vi "Measurement_input_panel.vi"(0 "OK":T4, 2 "setup":T5, 5 "Setup filename":string) -> (11 "Setup filename out":string, 12 "Analysis Info cluster":T8[](array[typedef])=[{"Colour"=0, "Inst type"=enum."Pitot-static tube", "Inst name"="Manometer voltage", "Symbol"="U", "Code name"="", "Extra Info"="U", "Inst Array"=enum."PWA", "Index"=0, "Voltage Index"=0, "Extra Titles"=[], "Extra Values"=[]}, {"Colour"=0, "Inst type"=enum."Pitot-static tube", "Inst name"="Manometer voltage", "Symbol"="U", "Code name"="", "Extra Info"="U", "Inst Array"=enum."PWA", "Index"=0, "Voltage Index"=0, "Extra Titles"=[], "Extra Values"=[]}, {"Colour"=0, "Inst type"=enum."Pitot-static tube", "Inst name"="Manometer voltage", "Symbol"="U", "Code name"="", "Extra Info"="U", "Inst Array"=enum."PWA", "Index"=0, "Voltage Index"=0, "Extra Titles"=[], "Extra Values"=[]}], 19 "Board type":T10=enum."Local ADAM")   [LabVIEW 2010]
uses:
  Controls/Inst_type.ctl
  Controls/Board_Types.ctl
  Controls/Analysis_info_cluster.ctl
  Controls/Instrument_Array.ctl
  Controls/Setup.ctl
  Controls/ok_button.ctl
  Controls/Trigger_Mode.ctl
  Controls/PWA_Data.ctl
  File/Setup_Filetype.ctl
  Controls/Post_Process.ctl
  Controls/App_Global.ctl
  Controls/Ch_and_Spans.ctl
  Globals/Meas_global.vi
  Globals/Trav_pos_global.vi
  Globals/LDA_meas_global_1.vi
  Globals/Preference_global.vi
panel:
  in  "Select Duplicate Channels":bool
  in  "PWA Data":T1
  out "Inst type":T2
  in  "Edit temp and Press":bool
  out "Abs Press (mbar)":dbl=1013.0 format="%.1f"
  out "Temp (deg C)":dbl=21.0 format="%.1f"
  in  "Trigger mode":T3
  in  "Select Plug Ins":bool
  in  "Sync Delay Time (ms)":dbl=24.0 format="%.2f"
  out "XW Present?":bool
  out "Read Setup File?":bool
  out "Setup Paths":string[](array[string])
  in  "Select Local ADAM Channels":bool
  out "Local ADAM Channels":string[](array[string])
  in  "stop":bool
  out "Notes":string
  in  "Setup filename selector":u16(ring) items=["Current_Setup.xls", "pitot_1.xls", "Calib_Setup.xls"]
  in  "Synchronise Analogue channels with LDA":bool
  in  "LDA set up":T6={"dimensions"=enum."2D", "Arrival spacing"=FALSE, "Transit time"=FALSE}
  in  "LDA data":enum16{"No LDA data", "Take LDA data"}(ring)=enum."Take LDA data"
  in  "Cross wire":T7(ring)
  in  "Acquisition Method":T10=enum."Local ADAM"
  in  "No of Analogue inst":i32=1
  in  "Ch & spans choices":T11(array[cluster]) {"D" format="%.2f"; "Ch No" min=0; "low limit" min=-10 max=10 format="%.2f"; "high limit" min=-10 max=10 format="%.2f"}
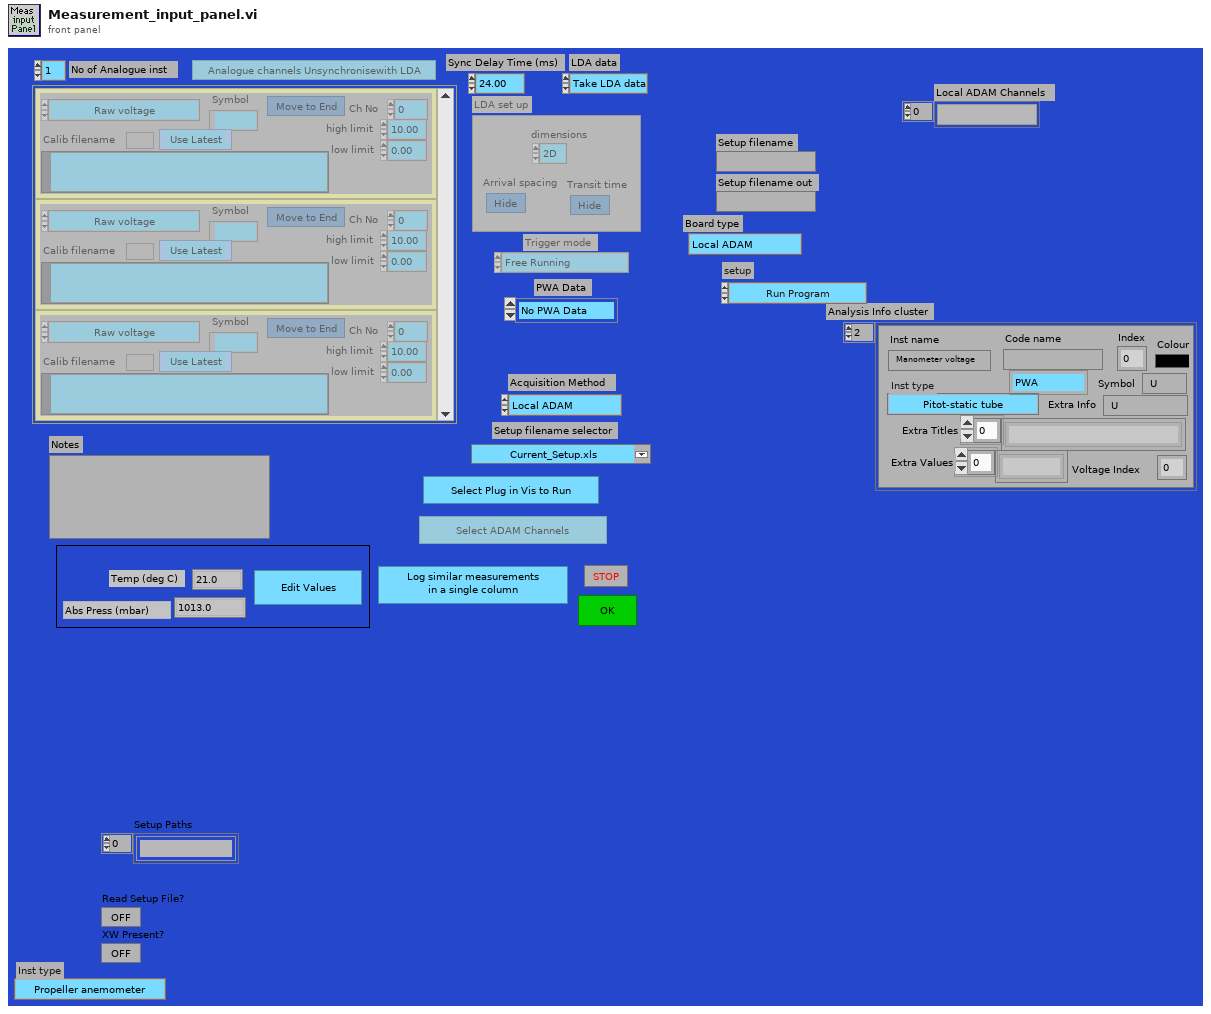
[diagram p1: front panel]
types:
  T1 = typedef "PWA_Data.ctl" = enum16{"No PWA Data", "One Ch PWA"}
  T2 = typedef "Inst_type.ctl" = enum16{"Propeller anemometer", "Raw voltage", "Pressure Transducer", "Pitot-static tube", "Preston tube", "Hot wire", "Cross wire 1", "Cross wire 2", "Generic Linear", "Generic Polynomial", "Generic BackPoly", "Fast FID", "Thermocouple", "Cold wire", "Pulsed Wire", "LDA Vel", "LDA Tran time", "LDA Arr time"}
  T3 = typedef "Trigger_Mode.ctl" = enum16{"Free Running", "Start on Trigger", "Trigger Every Block", "Trigger Every Sample"}
  T4 = typedef "ok_button.ctl" = bool
  T5 = typedef "Setup.ctl" = enum16{"Run Program", "Show Setup", "Save Current Setup", "Setup Front Panel"}
  T6 = cluster{"dimensions":enum16{"1D", "2D"}, "Arrival spacing":bool, "Transit time":bool}
  T7 = enum16{"2nd component as calculated", "2nd component multipled by -1"}
  T8 = typedef "Analysis_info_cluster.ctl" = cluster{"Colour":u32, "Inst type":T2, "Inst name":string, "Symbol":string, "Code name":string, "Extra Info":string, "Inst Array":T9, "Index":i32, "Voltage Index":i32, "Extra Titles":string[], "Extra Values":string[]}
  T9 = typedef "Instrument_Array.ctl" = enum16{"PWA", "LDA", "Analogue"}
  T10 = typedef "Board_Types.ctl" = enum16{"Simulate", "Local ADAM", "Server ADAM", "NI-DAQmx", "NI-DAQmxBase", "ADC488", "DT LV-link"}
  T11 = cluster{"high limit":sgl, "low limit":sgl, "Ch No":i16, "Calib filename":path, "Inst type":T2, "Symbol":string, "Move channel":bool, "Use Latest":bool, "D":dbl, "Ch Name":string}[]
  T12 = typedef "Post_Process.ctl" = enum16{"Take New Data", "Post Process Raw Data File"}
  T13 = typedef "Setup_Filetype.ctl" = enum16{"Measurement Setups", "Calibration Setups", "General", "Results File Plotter Setups", "Speed Calib Tweaks"}
  T14 = cluster{"high limit (10V)":sgl, "low limit (-10V)":sgl, "Ch No":i16, "Calib filename":path, "Inst type":T2, "Symbol":string, "Move channel":bool, "Use Latest":bool, "D":dbl, "Ch Name":string}
  T15 = typedef "App_Global.ctl" = enum16{"Read Global", "Write to Global", "Initialise Array"}
  T16 = typedef "Ch_and_Spans.ctl" = cluster{"high limit (10V)":sgl, "low limit (-10V)":sgl, "Ch No":i16, "Var name":string, "Use Latest Calib":bool}
  T17 = enum16{"Zero or one", "One", "Zero or more", "One or more"}
  T18 = enum8{"Enabled", "Disabled", "Disabled and Grayed Out"}
  T19 = typedef "Traverse_cluster.ctl" = cluster{"Start X":dbl, "Start Y":dbl, "Start Z":dbl, "End X":dbl, "End Y":dbl, "End Z":dbl, "No. of pts.":i32, "Spacing":T20, "Filename":path, "Tunnel Speed":dbl, "Averaging time (min)":dbl, "Extra Commands":string, "Specific Arguments":string, "Emission Rate (l/min)":dbl, "Trace Gas Concentration (%)":dbl, "Density Ratio":string, "Comments":string, "Row No":i32, "Row Type Selector":T21, "Completion time":string, "Row Duration (mins)":dbl, "No. of Valid pts.":i32, "Meas Setup File":string}
  T20 = typedef "Spacing.ctl" = enum16{"Linear", "Log", "Gauss", "Specified", "N/A"}
  T21 = typedef "Multi_run_mode.ctl" = enum16{"Move Traverse Only", "Set Tunnel Speed Only", "Set Source Only", "Set Measurement Conditions", "Single Measurement", "Vertical Profile", "Lateral Profile", "Longitudinal Profile", "Explore Volume", "Multi-Axis Profile", "Auto Calibrate", "Meas Fast FID Bkgnd", "Check Beam Power", "Scanning Valve Measurement", "Run VI Named:", "Set ADAM Ch", "Wait (minutes)", "Send Message", "Synchronize With:", "Fall Back to this Row", "Turn Off Row Repeating", "Blank Row"}
  T22 = cluster{"high limit (10V)":sgl, "low limit (-10V)":sgl, "Ch No":i16, "Calib filename":path, "Inst type":T2, "Symbol":string, "Move channel":bool, "Use Latest":bool, "D":dbl, "Ch Name":string}[]
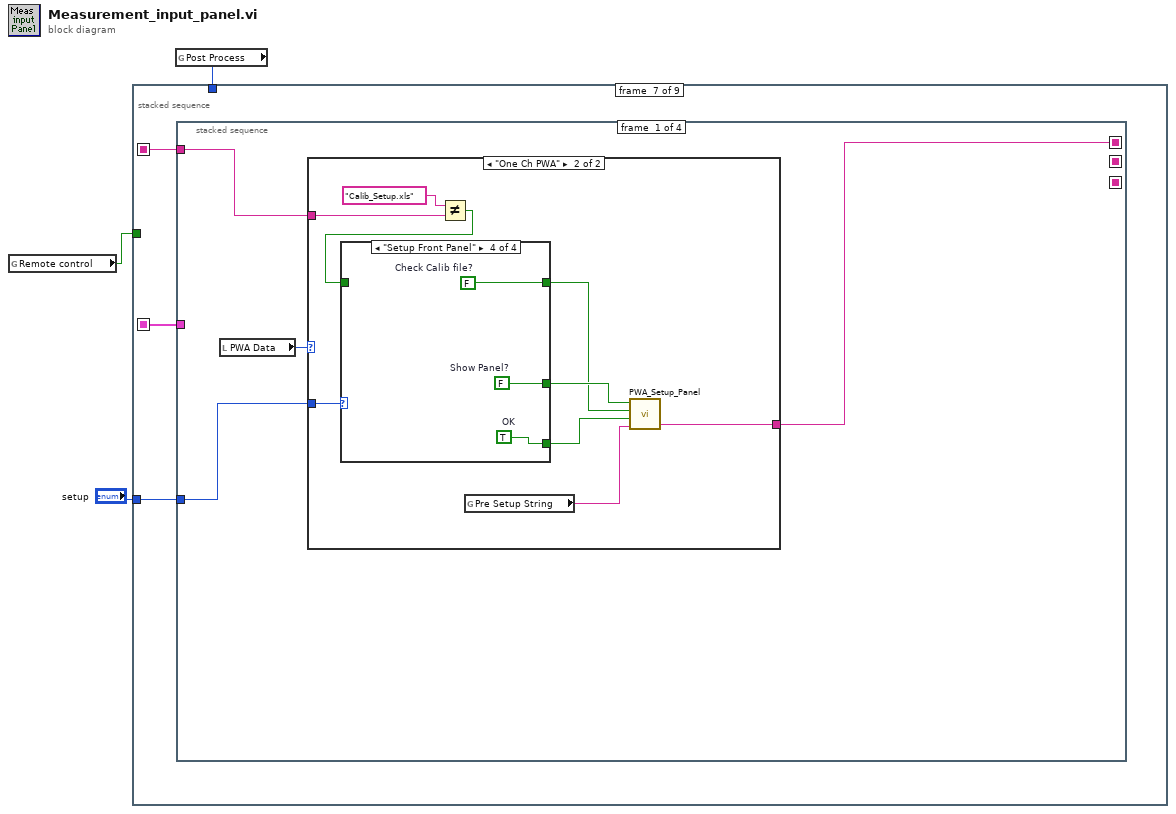
[diagram p0: block diagram]
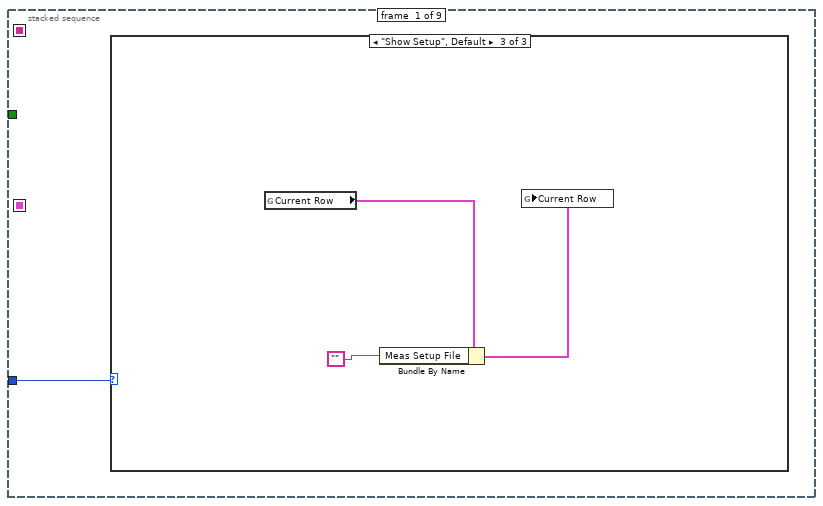
[diagram p2: hidden frame]
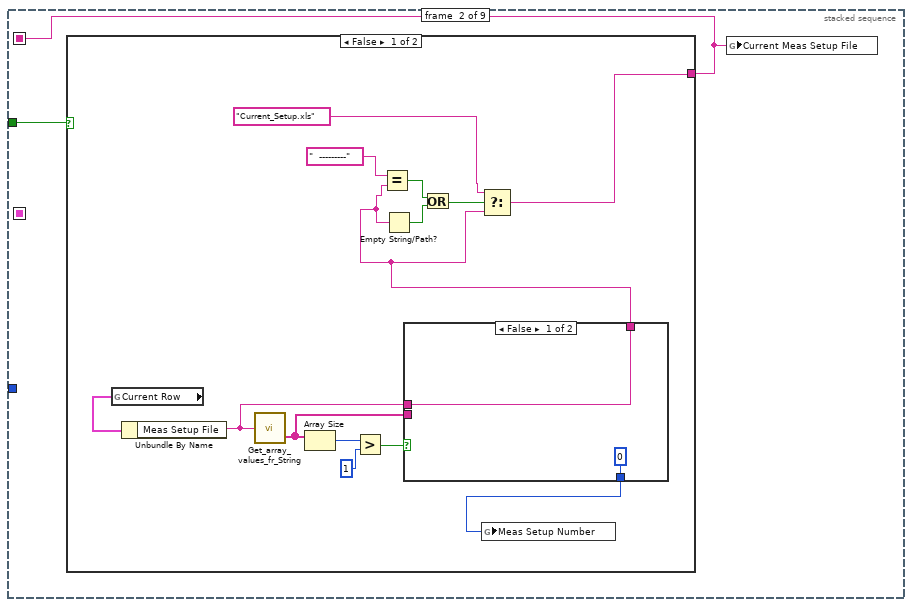
[diagram p5: hidden frame]
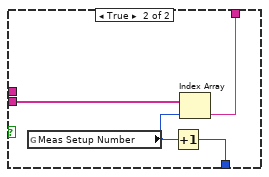
[diagram p6: hidden frame]
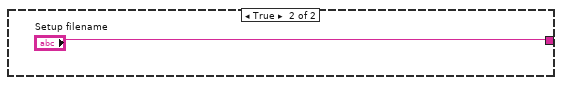
[diagram p7: hidden frame]
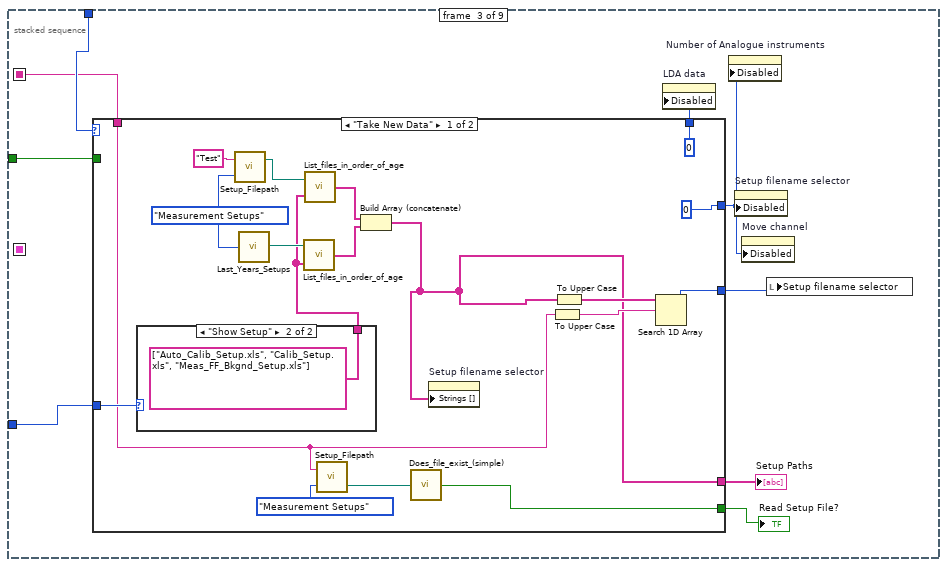
[diagram p8: hidden frame]
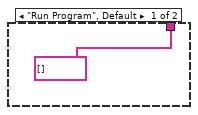
[diagram p9: hidden frame]
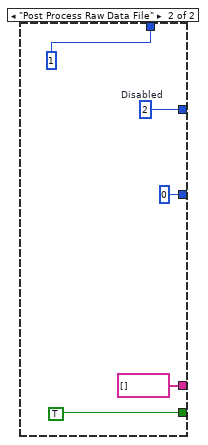
[diagram p10: hidden frame]
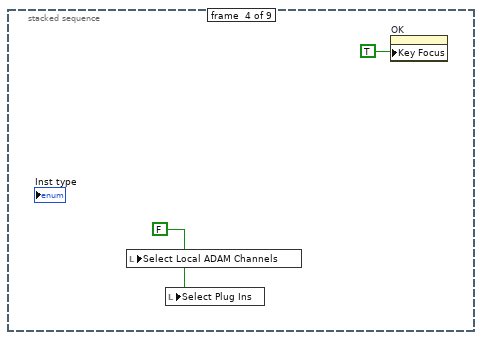
[diagram p11: hidden frame]
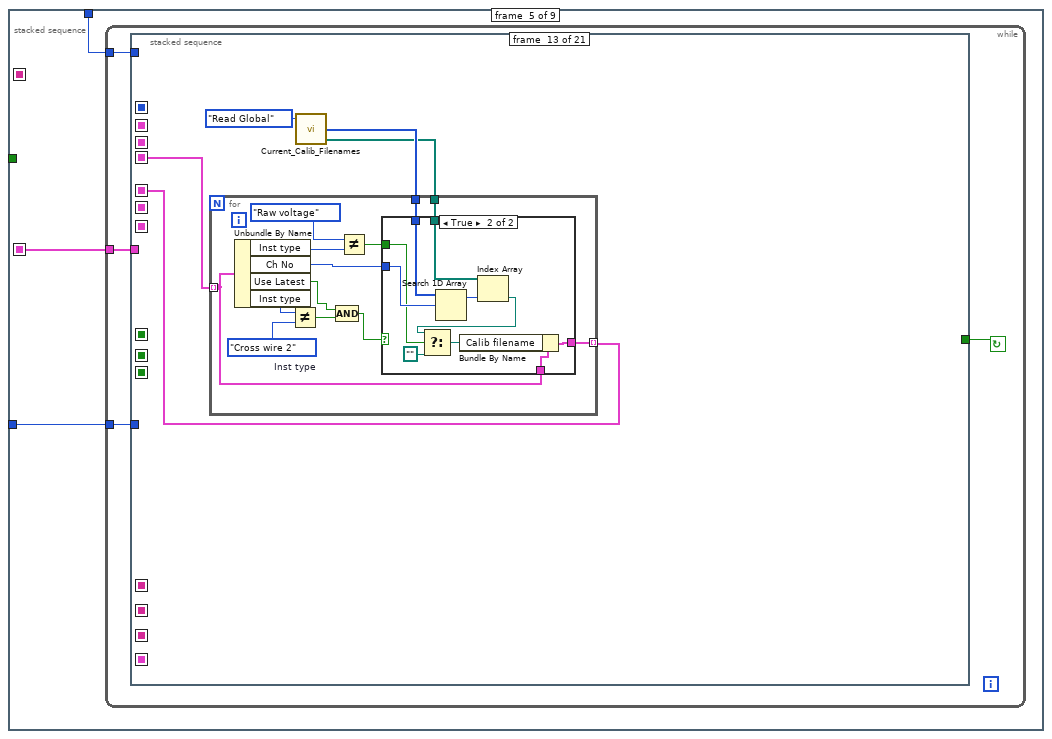
[diagram p12: hidden frame]
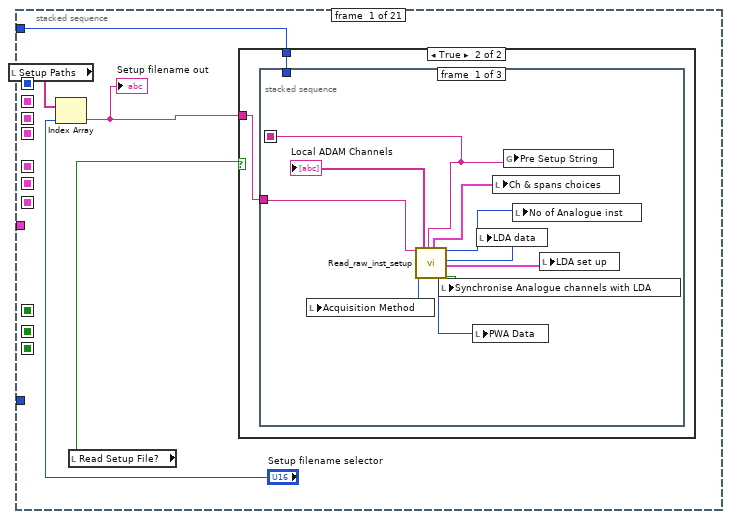
[diagram p13: hidden frame]
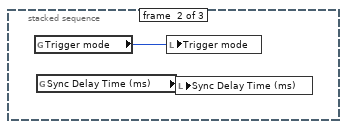
[diagram p15: hidden frame]
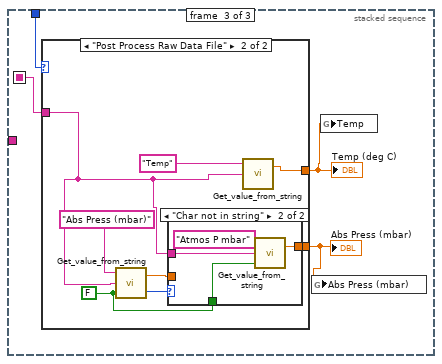
[diagram p16: hidden frame]
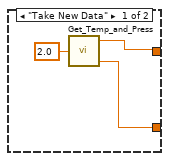
[diagram p17: hidden frame]
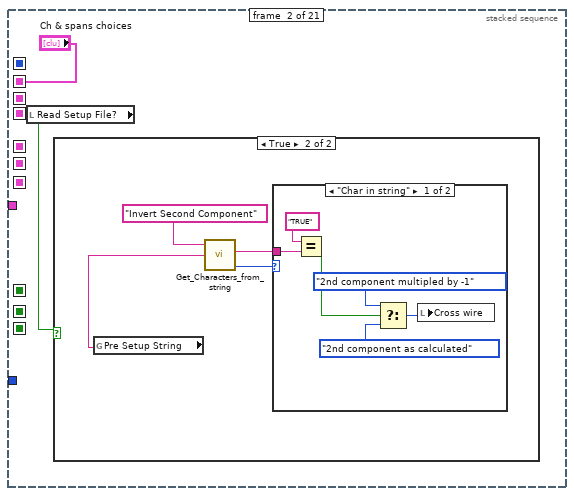
[diagram p19: hidden frame]
diagram:
  n1 = global read "Meas_global.vi" "Remote control"() -> (w1:bool)
  n2 = global read "Meas_global.vi" "Post Process"() -> (w3:T12)
  n3 = stacked-sequence {
    seq-local: [_ _ _ _ w69 _ _ _ _] -> [_ _ _ _ _ _ w723 _ w847]
    seq-local: [_ w8 _ _ _ _ _ _ _] -> [_ _ w31 _ _ _ w722 _ _]
    tunnel: w3 -> [_ _ w39 _ w68 _ _ _ w846]
    tunnel: "setup" -> [w4 _ w33 _ w67 _ w724 _ _]
    tunnel: w1 -> [_ w9 w32 _ _ _ _ _ _]
    frame #0 {
      n4 = case shown="\"Show Setup\", Default" w4 {
        frame "Run Program" {
        }
        frame "Setup Front Panel" {
        }
        frame "Show Setup", Default {
          n5 = global read "Trav_pos_global.vi" "Current Row"() -> (w7:T19)
          n6 = Bundle By Name(cluster=w7, "Meas Setup File"="") -> (w6:T19)
          n7 = global write "Trav_pos_global.vi" "Current Row"(w6) -> ()
        }
      }
    }
    frame #1 {
      n8 = case shown="False" w9 {
        tunnel: [w22 "Setup filename"] -> w8
        frame False {
          n9 = global read "Trav_pos_global.vi" "Current Row"() -> (w18:T19)
          n10 = Unbundle By Name(w18) -> ("Meas Setup File"=w12:string)
          n11 = call "Get_array_values_fr_String.vi"("String Value"=w12) -> ("String array"=w11:string[])  [unwired: 1 out]
          n12 = Array Size(array=w11) -> (size(s)=w16:i32)
          n13 = Greater?(x=w16, y=1) -> (0:w14:bool)
          n14 = case shown="False" w14 {
            tunnel: [w25 w28] -> w13
            tunnel: w12 -> [w25 _]
            tunnel: w11 -> [_ w29]
            tunnel: [0 w26] -> w10
            frame False {
            }
            frame True {
              n15 = global read "Trav_pos_global.vi" "Meas Setup Number"() -> (w27:i32)
              n16 = Increment(x=w27) -> (x+1=w26:i32)
              n17 = Index Array(array=w29, index=w27) -> (element=w28:string)
            }
          }
          n18 = Equal?(x="  ---------" ("f"), y=w13) -> (x = y?=w21:bool)
          n19 = Empty String/Path?(string/path=w13) -> (empty?=w20:bool)
          n20 = Or(x=w21, y=w20) -> (x .or. y?=w17:bool)
          n21 = Select(t="Current_Setup.xls", s=w17, f=w13) -> (s? t:f=w22:string)
          n22 = global write "Trav_pos_global.vi" "Meas Setup Number"(w10) -> ()
        }
        frame True {
        }
      }
      n23 = global write "Trav_pos_global.vi" "Current Meas Setup File"(w8) -> ()
    }
    frame #2 {
      n24 = case shown="\"Take New Data\"" w39 {
        tunnel: [w40 string[] []] -> w35
        tunnel: [w53 TRUE ("exists")] -> w34
        tunnel: [u8 0 ("Disabled") w61] -> w36
        tunnel: [u8 0 ("Disabled") u8 1 ("Disabled")] -> w38
        tunnel: w31 -> [w49 _]
        tunnel: [w56 0 ("index of element")] -> w37
        tunnel: w33 -> [w51 _]
        tunnel: w32 -> [_ _]
        frame "Take New Data" {
          w43 = Setup_Filetype."Measurement Setups" ("Setup File Type")
          n25 = case shown="\"Show Setup\"" w51 {
            tunnel: [string[] [] ("file names") string[] ["Auto_Calib_Setup.xls", "Calib_Setup.xls", "Meas_FF_Bkgnd_Setup.xls"] ("file names")] -> w41
            frame "Run Program", Default {
            }
            frame "Show Setup" {
            }
          }
          n26 = call "Setup_Filepath.vi"("Setup File Type"=w43, "Filename in"="Test") -> ("Directory"=w44:path)  [unwired: 1 out]
          n27 = call "Last_Years_Setups.vi"("Setup File Type"=w43) -> ("Directory"=w42:path)
          n28 = call "List_files_in_order_of_age.vi"("Files to Hide"=w41, "Folder"=w42) -> ("file names"=w46:string[])
          n29 = call "List_files_in_order_of_age.vi"("Files to Hide"=w41, "Folder"=w44) -> ("file names"=w45:string[])
          n30 = call "Setup_Filepath.vi"("Setup File Type"=Setup_Filetype."Measurement Setups", "Filename in"=w49) -> ("Filename Out"=w48:path)  [unwired: 1 out]
          n31 = Build Array (concatenate)(w45, w46) -> (w40:string[])
          n32 = call "Does_file_exist_(simple).vi"("Pathname"=w48) -> ("exists?"=w53:bool)
          n33 = property on="Setup filename selector" class="Ring (strict)"("Strings []"=w40) -> ()  [unwired: 2 in, 2 out]
          n34 = To Upper Case(1:w49) -> (0:w54:string)
          n35 = To Upper Case(1:w40) -> (0:w55:string[])
          n36 = Search 1D Array(1D array=w55, element=w54) -> (index of element=w56:i32)  [unwired: 1 out]
        }
        frame "Post Process Raw Data File" {
          w61 = u8 2  # Disabled
        }
      }
      "Setup Paths" <- w35
      "Read Setup File?" <- w34
      n37 = property on="LDA data" class="Enum (strict)"("Disabled"=w38) -> ()  [unwired: 2 in, 2 out]
      n38 = property on="Number of Analogue instruments" class="DigNum (strict)"("Disabled"=w36) -> ()  [unwired: 2 in, 2 out]
      n39 = property on="Setup filename selector" class="Ring (strict)"("Disabled"=w36) -> ()  [unwired: 2 in, 2 out]
      n40 = property on="Move channel" class="Bool (strict)"("Disabled"=w36) -> ()  [unwired: 2 in, 2 out]
      n41 = local write "Setup filename selector"(w37) -> ()
    }
    frame #3 {
      w66 = FALSE ("Select Local ADAM Channels")
      n42 = local write "Select Local ADAM Channels"(w66) -> ()
      n43 = local write "Select Plug Ins"(w66) -> ()
      n44 = property on="OK" class="Bool"("Key Focus"=TRUE) -> ()  [unwired: 2 in, 2 out]
    }
    frame #4 {
      n45 = while {
        tunnel: w67 -> [w70]
        tunnel: w68 -> [w71]
        tunnel: [w73] -> w69
        stop <- w72 continue-if-true
        n46 = stacked-sequence {
          seq-local: [_ _ _ _ _ _ _ _ w258 _ _ _ _ _ _ _ _ _ _ _ _] -> [_ _ _ _ _ _ _ _ _ _ w331 w376 w421 _ _ _ _ _ _ _ _]
          seq-local: [_ _ _ w147 _ _ _ _ _ _ _ _ _ _ _ _ _ _ _ _ _] -> [_ _ _ _ _ w200 w235 w254 w259 _ _ _ _ _ _ _ _ _ _ _ _]
          seq-local: [_ _ _ _ _ w205 _ _ _ _ _ _ _ _ _ _ _ _ _ _ _] -> [_ _ _ _ _ _ _ _ w260 _ _ _ _ _ _ _ _ _ _ _ _]
          seq-local: [_ _ _ _ _ _ _ _ _ _ w333 _ _ _ _ _ _ _ _ _ _] -> [_ _ _ _ _ _ _ _ _ _ _ w378 _ _ _ _ _ _ _ _ w684]
          seq-local: [_ _ _ _ _ _ _ _ _ _ _ _ _ w454 _ _ _ _ _ _ _] -> [_ _ _ _ _ _ _ _ _ _ _ _ _ _ w473 _ _ _ _ _ _]
          seq-local: [_ _ _ _ _ _ _ _ _ _ _ _ _ _ w469 _ _ _ _ _ _] -> [_ _ _ _ _ _ _ _ _ _ _ _ _ _ _ w495 w501 w564 _ w657 w685]
          seq-local: [_ _ _ _ _ _ _ _ _ _ _ w382 _ _ _ _ _ _ _ _ _] -> [_ _ _ _ _ _ _ _ _ _ _ _ _ w451 _ _ _ _ _ _ _]
          seq-local: [_ _ _ _ _ _ _ _ _ _ _ _ w425 _ _ _ _ _ _ _ _] -> [_ _ _ _ _ _ _ _ _ _ _ _ _ w450 _ _ _ _ _ _ _]
          seq-local: [_ _ _ _ _ _ _ _ _ w318 _ _ _ _ _ _ _ _ _ _ _] -> [_ _ _ _ _ _ _ _ _ _ w332 w379 _ _ _ _ _ _ _ _ w683]
          seq-local: [_ _ _ _ _ _ _ _ _ _ _ _ _ _ _ _ w500 _ _ _ _] -> [_ _ _ _ _ _ _ _ _ _ _ _ _ _ _ _ _ w567 _ _ _]
          seq-local: [_ _ _ _ _ _ _ _ _ _ _ _ _ _ _ _ w499 _ _ _ _] -> [_ _ _ _ _ _ _ _ _ _ _ _ _ _ _ _ _ w566 _ _ _]
          seq-local: [_ _ _ _ _ _ _ _ _ _ _ _ _ _ _ _ w498 _ _ _ _] -> [_ _ _ _ _ _ _ _ _ _ _ _ _ _ _ _ _ w565 _ _ _]
          seq-local: [_ _ _ _ _ _ _ _ _ _ _ _ _ _ _ _ _ w563 _ _ _] -> [_ _ _ _ _ _ _ _ _ _ _ _ _ _ _ _ _ _ w605 _ _]
          seq-local: [_ "Ch & spans choices" _ _ _ _ _ _ _ _ _ _ _ _ _ _ _ _ _ _ _] -> [_ _ _ w134 _ _ _ _ _ _ _ _ _ _ _ w494 _ _ _ _ _]
          tunnel: [_ _ _ _ _ _ _ _ _ _ _ _ _ _ w469 _ _ _ _ _ _] -> w73
          tunnel: [_ _ _ _ _ _ _ _ _ _ _ w380 _ _ _ _ _ _ _ _ _] -> w72
          tunnel: w71 -> [w75 _ w125 w142 _ _ _ _ _ w319 _ w377 _ w453 _ _ _ _ _ w658 _]
          tunnel: w70 -> [_ _ _ _ w186 _ _ _ _ _ _ _ _ w452 _ _ _ _ w607 _ _]
          frame #0 {
            n47 = local read "Setup Paths"() -> (w78:string[])
            n48 = Index Array(array=w78, index="Setup filename selector") -> (element=w74:string)
            "Setup filename out" <- w74
            n49 = local read "Read Setup File?"() -> (w77:bool)
            n50 = case shown="True" w77 {
              tunnel: w74 -> [_ w80]
              tunnel: w75 -> [_ w79]
              frame False {
              }
              frame True {
                n51 = stacked-sequence {
                  seq-local: [w83 _ _] -> [_ _ w95]
                  tunnel: w80 -> [w86 _ _]
                  tunnel: w79 -> [_ _ w96]
                  frame #0 {
                    n52 = call "Read_raw_inst_setup.vi"("Setup file"=w86) -> ("Board type"=w88:T10, "Local ADAM Channels"=→"Local ADAM Channels":string[], "Setup string"=w83:string, "Ch & spans choices"=w82:T22, "PWA Data"=w81:T1, "Number of Analogue instruments"=w90:i32, "LDA data"=w89:enum16{"No LDA data", "Take LDA data"}, "LDA set up"=w85:T6, "Synchronise Analogue channels with LDA"=w87:bool)  [unwired: 10 out]
                    n53 = local write "Acquisition Method"(w88) -> ()
                    n54 = local write "Synchronise Analogue channels with LDA"(w87) -> ()
                    n55 = local write "PWA Data"(w81) -> ()
                    n56 = local write "LDA data"(w89) -> ()
                    n57 = local write "Ch & spans choices"(w82) -> ()
                    n58 = global write "Meas_global.vi" "Pre Setup String"(w83) -> ()
                    n59 = local write "No of Analogue inst"(w90) -> ()
                    n60 = local write "LDA set up"(w85) -> ()
                  }
                  frame #1 {
                    n61 = global read "Meas_global.vi" "Trigger mode"() -> (w91:T3)
                    n62 = global read "LDA_meas_global_1.vi" "Sync Delay Time (ms)"() -> (w92:dbl)
                    n63 = local write "Trigger mode"(w91) -> ()
                    n64 = local write "Sync Delay Time (ms)"(w92) -> ()
                  }
                  frame #2 {
                    n65 = case shown="\"Post Process Raw Data File\"" w96 {
                      tunnel: w95 -> [_ w102]
                      tunnel: [w97 w101] -> w93
                      tunnel: [w98 w100] -> w94
                      frame "Take New Data" {
                        n66 = call "Get_Temp_and_Press.vi"("Averaging time (mins)"=2.0) -> ("Abs Press (mbar)"=w97:dbl, "Temperature"=w98:dbl)  [unwired: 3 out]
                      }
                      frame "Post Process Raw Data File" {
                        w104 = FALSE ("Show Dialog?")
                        n67 = call "Get_value_from_string.vi"("Show Dialog?"=w104, "Input string"=w102, "Variable name"="Abs Press (mbar)") -> ("Status"=w106:enum16{"Char in string", "Char not in string"}, "Value"=w105:dbl)
                        n68 = case shown="\"Char not in string\"" w106 {
                          tunnel: [w108 w111] -> w101
                          tunnel: w105 -> [w108 _]
                          tunnel: w104 -> [_ w110]
                          tunnel: w102 -> [_ w109]
                          frame "Char in string" {
                          }
                          frame "Char not in string" {
                            n69 = call "Get_value_from_string.vi"("Show Dialog?"=w110, "Input string"=w109, "Variable name"="Atmos P mbar") -> ("Value"=w111:dbl)  [unwired: 1 out]
                          }
                        }
                        n70 = call "Get_value_from_string.vi"("Input string"=w102, "Variable name"="Temp") -> ("Value"=w100:dbl)  [unwired: 1 in, 1 out]
                      }
                    }
                    "Abs Press (mbar)" <- w93
                    "Temp (deg C)" <- w94
                    n71 = global write "Meas_global.vi" "Abs Press (mbar)"(w93) -> ()
                    n72 = global write "Meas_global.vi" "Temp"(w94) -> ()
                  }
                }
              }
            }
          }
          frame #1 {
            n73 = local read "Read Setup File?"() -> (w114:bool)
            n74 = case shown="True" w114 {
              frame False {
              }
              frame True {
                n75 = global read "Meas_global.vi" "Pre Setup String"() -> (w117:string)
                n76 = call "Get_Characters_from_string.vi"("Input string"=w117, "Variable name"="Invert Second Component") -> ("Status"=w116:enum16{"Char in string", "Char not in string"}, "Value"=w115:string)  [unwired: 1 in]
                n77 = case shown="\"Char in string\"" w116 {
                  tunnel: w115 -> [w124 _]
                  frame "Char in string" {
                    n78 = Equal?(x="TRUE", y=w124) -> (x = y?=w120:bool)
                    n79 = Select(t=T7."2nd component multipled by -1" ("Cross wire/LDA"), s=w120, f=T7."2nd component as calculated" ("Cross wire/LDA")) -> (s? t:f=w122:T7)
                    n80 = local write "Cross wire"(w122) -> ()
                  }
                  frame "Char not in string" {
                  }
                }
              }
            }
          }
          frame #2 {
            n81 = case shown="True" "Edit temp and Press" {
              tunnel: w125 -> [_ w127]
              frame False {
              }
              frame True {
                n82 = case shown="\"Take New Data\"" w127 {
                  frame "Take New Data" {
                    n83 = stacked-sequence {
                      frame #0 {
                        w128 = TRUE  # Wait until done
                        n84 = call "Run_Enter_Temp.vi"("Wait until done"=w128) -> ()  [unwired: 1 out]
                      }
                      frame #1 {
                        n85 = call "Get_Temp_and_Press.vi"("Averaging time (mins)"=2.0) -> ("Abs Press (mbar)"=w129:dbl, "Temperature"=w130:dbl)  [unwired: 3 out]
                        n86 = local write "Temp (deg C)"(w130) -> ()
                        n87 = local write "Abs Press (mbar)"(w129) -> ()
                      }
                    }
                  }
                  frame "Post Process Raw Data File" {
                  }
                }
              }
            }
          }
          frame #3 {
            w138 = u8 0  # Disabled
            n88 = local read "Read Setup File?"() -> (w133:bool)
            n89 = Equal?(x=w142, y=Post_Process."Take New Data" ("Post Process")) -> (x = y?=w141:bool)
            n90 = local read "Acquisition Method"() -> (w135:T10)
            n91 = Equal?(x=w135, y=Board_Types."Local ADAM" ("Board type")) -> (x = y?=w132:bool)
            n92 = And(x=w133, y=w132) -> (x .and. y?=w146:bool)
            n93 = Or(x="Select Local ADAM Channels", y=w146) -> (x .or. y?=w139:bool)
            n94 = And(x=w141, y=w139) -> (x .and. y?=w140:bool)
            n95 = case shown="True" w140 {
              tunnel: [w149 w152] -> w147
              tunnel: w134 -> [w149 w153]
              tunnel: "Select Local ADAM Channels" -> [_ w151]
              tunnel: w132 -> [_ w150]
              frame False {
              }
              frame True {
                n96 = local read "Local ADAM Channels"() -> (w155:string[])
                n97 = stacked-sequence {
                  seq-local: [_ w164 _ _ _] -> [_ _ w170 w183 _]
                  seq-local: [_ w168 _ _ _] -> [_ _ w174 _ _]
                  seq-local: [T14 {"high limit (10V)"=10.0, "low limit (-10V)"=0.0, "Ch No"=0, "Calib filename"=path "", "Inst type"=enum."Raw voltage", "Symbol"="", "Move channel"=FALSE, "Use Latest"=FALSE, "D"=0.0, "Ch Name"=""} _ _ _ _] -> [_ w160 _ _ _]
                  seq-local: [_ w157 _ _ _] -> [_ _ w172 _ _]
                  tunnel: w155 -> [_ w167 _ _ _]
                  tunnel: [_ w168 _ _ _] -> w154
                  tunnel: w153 -> [_ w159 _ _ _]
                  tunnel: [_ _ w173 _ _] -> w152
                  tunnel: w151 -> [_ w169 _ _ w184]
                  tunnel: w150 -> [_ w165 w171 _ _]
                  frame #0 {
                  }
                  frame #1 {
                    n98 = Array Size(array=w159) -> (size(s)=w162:i32)
                    n99 = Array Subset(array=w167, length=w162) -> (w166:string[])  [unwired: 1 in]
                    n100 = call "Get_local_ADAM_Chs.vi"("Local ADAM?"=w165, "Show setup"=w169, "Desired Local ADAM Channels"=w166) -> ("Choosen Channels"=w168:string[], "Ch Indicies Choosen"=w164:i32[])
                    n101 = Array Size(array=w164) -> (size(s)=w163:i32)
                    n102 = Subtract(x=w163, y=w162) -> (x-y=w161:i32)
                    n103 = Initialize Array(w160, w161) -> (w158:T22)
                    n104 = Build Array (concatenate)(w159, w158) -> (w157:T22)
                  }
                  frame #2 {
                    n105 = for {
                      tunnel: [w181] -> w173 mode=indexing
                      tunnel: w174 -> [w180] mode=indexing
                      tunnel: w172 -> [w179] mode=indexing
                      tunnel: w171 -> [w178]
                      tunnel: w170 -> [w177] mode=indexing
                      i -> [w176]
                      n106 = Select(t=w177, s=w178, f=w176) -> (s? t:f=w175:i32)
                      n107 = Bundle By Name(cluster=w179, "Ch No"=w175, "Ch Name"=w180) -> (w181:T14)
                    }
                  }
                  frame #3 {
                    n108 = Array Size(array=w183) -> (size(s)=w182:i32)
                    n109 = local write "No of Analogue inst"(w182) -> ()
                  }
                  frame #4 {
                    n110 = case shown="True" w184 {
                      frame False {
                      }
                      frame True {
                        n111 = local write "Select Local ADAM Channels"(FALSE ("Select Local ADAM Channels")) -> ()
                      }
                    }
                  }
                }
                n112 = local write "Local ADAM Channels"(w154) -> ()
              }
            }
            n113 = Select(t=w138, s=w132, f=u8 2 ("Disabled")) -> (s? t:f=w136:u8)
            n114 = property on="Ch Name" class="Str"("Visible"=w132) -> ()  [unwired: 2 in, 2 out]
            n115 = property on="Select Local ADAM Channels" class="Bool (strict)"("Disabled"=w136) -> ()  [unwired: 2 in, 2 out]
            n116 = Not(x=w132) -> (.not. x?=w144:bool)
            n117 = property on="high limit" class="DigNum (strict)"("Visible"=w144) -> ()  [unwired: 2 in, 2 out]
            n118 = property on="low limit" class="DigNum (strict)"("Visible"=w144) -> ()  [unwired: 2 in, 2 out]
          }
          frame #4 {
            n119 = case shown="True" "Select Plug Ins" {
              tunnel: w186 -> [_ w188]
              frame False {
              }
              frame True {
                n120 = stacked-sequence {
                  tunnel: w188 -> [w189 _]
                  frame #0 {
                    w193 = TRUE  # Show Panel?
                    n121 = global read "Meas_global.vi" "Pre Setup String"() -> (w192:string)
                    n122 = local write "Select Plug Ins"(FALSE ("Select Local ADAM Channels")) -> ()
                    n123 = call "Choose_Plug_In_to_Run.vi"("setup"=w189, "Show Panel?"=w193, "Setup String In"=w192) -> ("Setup String Out"=w191:string)  [unwired: 1 out]
                    n124 = global write "Meas_global.vi" "Pre Setup String"(w191) -> ()
                  }
                  frame #1 {
                    n125 = Current VI's Path() -> (path=w195:path)
                    n126 = call "Open_Close_Front_Panel.ph.vi"("Front Panel Window:Open"=TRUE, "VI path"=w195) -> ()  [unwired: 2 out]
                  }
                }
              }
            }
          }
          frame #5 {
            n127 = Initialize Array(0) -> (w207:i32[])  [unwired: 1 out]
            n128 = for {
              shift-right: [w214] -> w203
              shift-left: w207 -> [w215]
              tunnel: [w213] -> w201 mode=indexing
              tunnel: w200 -> [w212] mode=indexing
              tunnel: [w210] -> w199 mode=indexing
              n129 = Unbundle By Name(w212) -> ("Inst type"=w209:T2)
              n130 = case shown="\"Cross wire 1\"" w209 {
                tunnel: w215 -> [w219 w223 w225 w229]
                tunnel: [w218 w222 w225 w228] -> w214
                tunnel: [FALSE TRUE FALSE FALSE] -> w213
                frame "Propeller anemometer", Default {
                  n131 = Build Array (concatenate)(w219, 1) -> (w218:i32[])
                }
                frame "Cross wire 1" {
                  n132 = Build Array (concatenate)(w223, 2) -> (w222:i32[])
                }
                frame "Cross wire 2" {
                }
                frame "LDA Vel" {
                  n133 = Build Array (concatenate)(w229, 1) -> (w228:i32[])
                }
              }
              n134 = Equal?(x=w209, y=Inst_type."Preston tube" ("Inst type")) -> (x = y?=w210:bool)
            }
            n135 = Build Array (concatenate)(w203, 1) -> (w202:i32[])
            n136 = Array Subset(array=w202, length="No of Analogue inst") -> (w206:i32[])  [unwired: 1 in]
            n137 = Add Array Elements(numeric array=w206) -> (sum=w205:i32)
            n138 = Or Array Elements(Boolean array=w201) -> (logical OR=→"XW Present?":bool)
            n139 = Or Array Elements(Boolean array=w199) -> (logical OR=w197:bool)
            n140 = property on="D" class="DigNum (strict)"("Visible"=w197) -> ()  [unwired: 2 in, 2 out]
          }
          frame #6 {
            n141 = local read "Acquisition Method"() -> (w233:T10)
            n142 = Equal?(x=w233, y=Board_Types."Local ADAM" ("Board type")) -> (x = y?=w231:bool)
            n143 = for {
              tunnel: w235 -> [w240] mode=indexing
              shift-right: [w238] -> w230
              shift-left: "" -> [w237]
              tunnel: w231 -> [w236]
              n144 = Unbundle By Name(w240) -> ("Inst type"=w239:T2)
              n145 = case shown="\"Cross wire 1\"" w239 {
                tunnel: [w242 w249] -> w238
                tunnel: w237 -> [w243 w249]
                tunnel: w236 -> [w241 _]
                frame "Cross wire 1" {
                  n146 = case shown="True" w241 {
                    tunnel: w243 -> [w244 w248]
                    tunnel: [w244 w247] -> w242
                    frame False {
                    }
                    frame True {
                      n147 = Concatenate Strings(w248, "WARNING!\nCheck that sample and hold is working for the cross wire channels. It will affect your results!\n", "\r\n") -> (w247:string)
                    }
                  }
                }
                frame "Generic Linear", Default {
                }
              }
            }
            "Notes" <- w230
          }
          frame #7 {
            n148 = local read "Acquisition Method"() -> (→"Board type":T10)
            n149 = Array Size(array=w254) -> (size(s)=w253:i32)
            n150 = Not Equal To 0?(x=w253) -> (x != 0?=w252:bool)
            n151 = case shown="True" w252 {
              tunnel: [enum16{"No Analogue data", "Take Analogue data"}."No Analogue data" ("Analogue data") enum16{"No Analogue data", "Take Analogue data"}."Take Analogue data" ("Analogue data")] -> w251
              frame False {
              }
              frame True {
              }
            }
            n152 = global write "Meas_global.vi" "Analogue data"(w251) -> ()
          }
          frame #8 {
            n153 = Index Array(array=w259, index=0) -> (element=w264:T14)
            n154 = Initialize Array(w264) -> (w262:T22)  [unwired: 1 out]
            n155 = Build Array (concatenate)(w259, w264) -> (w263:T22)
            n156 = for {
              N: w260 -> [_]
              tunnel: w263 -> [w272] mode=indexing
              shift-right: [w273] -> w258
              shift-left: w262 -> [w267]
              tunnel: Inst_type."Cross wire 2" ("Inst type") -> [w265]
              shift-right: [w271] -> _
              shift-left: _ -> [w270]
              tunnel: w263 -> [w269]
              n157 = Unbundle By Name(w272) -> ("Inst type"=w271:T2)
              n158 = Array Size(array=w267) -> (size(s)=w266:i32)
              n159 = Increment(x=w266) -> (x+1=w268:i32)
              n160 = case shown="\"Cross wire 1\"" w271 {
                tunnel: [w282 w303 w315] -> w273
                tunnel: w267 -> [w283 w305 w317]
                tunnel: w272 -> [w279 w306 w316]
                tunnel: w265 -> [w281 w310 _]
                tunnel: w270 -> [_ w309 _]
                tunnel: w269 -> [w286 _ _]
                tunnel: w268 -> [w285 _ _]
                frame "Cross wire 1" {
                  n161 = Index Array(array=w286, index=w285) -> (element=w280:T14)
                  n162 = Unbundle By Name(w280) -> ("Inst type"=w284:T2, "high limit (10V)"=w277:sgl, "low limit (-10V)"=w276:sgl, "Ch No"=w275:i16, "Symbol"=w274:string)
                  n163 = Unbundle By Name(w279) -> ("Calib filename"=w278:path)
                  n164 = case shown="\"Generic Linear\", Default" w284 {
                    tunnel: w283 -> [w296 w302]
                    tunnel: [w295 w301] -> w282
                    tunnel: w281 -> [w288 w297]
                    tunnel: w278 -> [w294 w300]
                    tunnel: w279 -> [w292 w298]
                    tunnel: w280 -> [_ _]
                    tunnel: w277 -> [w291 _]
                    tunnel: w276 -> [w290 _]
                    tunnel: w275 -> [w289 _]
                    tunnel: w274 -> [w287 _]
                    frame "Cross wire 2" {
                      n165 = Bundle By Name(cluster=w292, "Calib filename"=w294, "Inst type"=w288, "high limit (10V)"=w291, "low limit (-10V)"=w290, "Ch No"=w289, "Symbol"=w287) -> (w293:T14)
                      n166 = Build Array (concatenate)(w296, w292, w293) -> (w295:T22)
                    }
                    frame "Generic Linear", Default {
                      n167 = Bundle By Name(cluster=w298, "Calib filename"=w300, "Inst type"=w297) -> (w299:T14)
                      n168 = Build Array (concatenate)(w302, w298, w299) -> (w301:T22)
                    }
                  }
                }
                frame "Cross wire 2" {
                  n169 = Decrement(x=w310) -> (x-1=w308:T2)
                  n170 = Equal?(x=w308, y=w309) -> (x = y?=w307:bool)
                  n171 = Bundle By Name(cluster=w306, "Inst type"=w308) -> (w304:T14)
                  n172 = case shown="False" w307 {
                    tunnel: w306 -> [_ _]
                    tunnel: w305 -> [w313 w314]
                    tunnel: w304 -> [w312 _]
                    tunnel: [w311 w314] -> w303
                    frame False {
                      n173 = Build Array (concatenate)(w313, w312) -> (w311:T22)
                    }
                    frame True {
                    }
                  }
                }
                frame "Generic Linear", Default {
                  n174 = Build Array (concatenate)(w317, w316) -> (w315:T22)
                }
              }
            }
          }
          frame #9 {
            n175 = case shown="\"Simulate\"" "Acquisition Method" {
              tunnel: [w324 w325 w326 w327 w328 w329 w330] -> w322
              tunnel: [w324 w325 w326 w327 w328 w329 w330] -> w321
              frame "Simulate" {
                w324 = TRUE
              }
              frame "Local ADAM" {
                w325 = FALSE
              }
              frame "Server ADAM" {
                w326 = FALSE
              }
              frame "NI-DAQmx" {
                w327 = TRUE
              }
              frame "NI-DAQmxBase" {
                w328 = TRUE
              }
              frame "ADC488" {
                w329 = TRUE
              }
              frame "DT LV-link" {
                w330 = TRUE
              }
            }
            n176 = Equal?(x=w319, y=Post_Process."Take New Data" ("Post Process")) -> (x = y?=w318:bool)
            n177 = property on="high limit" class="DigNum (strict)"("Visible"=w322) -> ()  [unwired: 2 in, 2 out]
            n178 = property on="low limit" class="DigNum (strict)"("Visible"=w321) -> ()  [unwired: 2 in, 2 out]
          }
          frame #10 {
            n179 = case shown="True" "OK" {
              tunnel: w331 -> [_ w348]
              tunnel: [FALSE w347] -> w333
              tunnel: w332 -> [_ w336]
              frame False {
              }
              frame True {
                n180 = for {
                  tunnel: w348 -> [w360] mode=indexing
                  tunnel: [w358] -> w342 mode=indexing
                  tunnel: [w354] -> w346 mode=indexing
                  n181 = Unbundle By Name(w360) -> ("high limit (10V)"=w363:sgl, "low limit (-10V)"=w362:sgl, "Ch No"=w359:i16, "Inst type"=w357:T2, "Symbol"=w356:string)
                  n182 = Number To Decimal String(number=w357) -> (decimal integer string=w355:string)  [unwired: 1 out]
                  n183 = Concatenate Strings(w355, w356) -> (w354:string)
                  n184 = Greater Or Equal?(x=w363, y=w362) -> (x >= y?=w361:bool)
                  n185 = case shown="\"Propeller anemometer\", Default" w357 {
                    tunnel: w361 -> [w366 _ _ _]
                    tunnel: w359 -> [w365 _ _ _]
                    tunnel: [w364 TRUE TRUE TRUE] -> w358
                    frame "Propeller anemometer", Default {
                      n186 = case shown="True" w366 {
                        tunnel: w365 -> [w369 _]
                        tunnel: [FALSE TRUE] -> w364
                        frame False {
                          n187 = Number To Decimal String(number=w369) -> (decimal integer string=w368:string)  [unwired: 1 out]
                          n188 = Concatenate Strings("Error in input limits for Channel No ", w368) -> (w370:string)
                          n189 = One Button Dialog(message=w370) -> ()  [unwired: 2 out]
                        }
                        frame True {
                        }
                      }
                    }
                    frame "LDA Vel" {
                    }
                    frame "LDA Tran time" {
                    }
                    frame "LDA Arr time" {
                    }
                  }
                }
                n190 = call "Analyse_string_array.vi"("String array"=w346) -> ("Frequency"=w345:i32[])  [unwired: 2 out]
                n191 = global read "Meas_global.vi" "Remote control"() -> (w337:bool)
                n192 = Greater?(x=w345, y=1) -> (0:w343:bool[])
                n193 = Or Array Elements(Boolean array=w343) -> (logical OR=w339:bool)
                n194 = Compound Arithmetic op=AND(invert w337, w339, w336) -> (w338:bool)
                n195 = case shown="True" w338 {
                  tunnel: [TRUE FALSE] -> w341
                  frame False {
                  }
                  frame True {
                    n196 = Current VI's Path() -> (path=w351:path)
                    n197 = call "Open_Close_Front_Panel.ph.vi"("Front Panel Window:Open"=TRUE, "VI path"=w351) -> ()  [unwired: 2 out]
                    n198 = One Button Dialog(message="Non Unique symbol names") -> ()  [unwired: 2 out]
                  }
                }
                n199 = Build Array (concatenate)(w342, w341) -> (w340:bool[])
                n200 = And Array Elements(Boolean array=w340) -> (logical AND=w347:bool)
              }
            }
          }
          frame #11 {
            n201 = And(x=w379, y=w378) -> (x .and. y?=w381:bool)
            n202 = case shown="True" w381 {
              tunnel: w376 -> [_ w389]
              tunnel: [FALSE w388] -> w382
              tunnel: [w383 w387] -> w380
              tunnel: w378 -> [w384 _]
              tunnel: w377 -> [_ _]
              frame False {
                n203 = Not(x=w384) -> (.not. x?=w383:bool)
              }
              frame True {
                n204 = for {
                  shift-right: [w408] -> _
                  shift-left: i16[] [] -> [w407]
                  tunnel: w389 -> [w404] mode=indexing
                  tunnel: [w395] -> w390 mode=indexing
                  shift-right: [w403] -> _
                  shift-left: path[] [] -> [w402]
                  n205 = Unbundle By Name(w404) -> ("Ch No"=w405:i16)
                  n206 = Unbundle By Name(w404) -> ("Inst type"=w401:T2, "Calib filename"=w398:path)
                  n207 = Search 1D Array(1D array=w407, element=w405) -> (index of element=w406:i32)  [unwired: 1 out]
                  n208 = Build Array (concatenate)(w407, w405) -> (w408:i16[])
                  n209 = Equal?(x=Inst_type."Fast FID" ("Inst type"), y=w401) -> (x = y?=w394:bool)
                  n210 = case shown="0, Default" w406 {
                    tunnel: w405 -> [w419 _]
                    tunnel: [w415 FALSE ("true")] -> w397
                    frame 0, Default {
                      n211 = Format Into String(format string="The Ch No %d appears more than once", w419) -> (resulting string=w417:string)  [unwired: 2 in, 1 out]
                      n212 = One Button Dialog(message=w417, button name ("OK")="Ok") -> (true=w415:bool)
                    }
                    frame -1 {
                    }
                  }
                  n213 = Search 1D Array(1D array=w402, element=w398) -> (index of element=w399:i32)  [unwired: 1 out]
                  n214 = Greater Or Equal To 0?(x=w399) -> (x >= 0?=w393:bool)
                  n215 = And(x=w394, y=w393) -> (x .and. y?=w392:bool)
                  n216 = case shown="True" w392 {
                    tunnel: [w410 FALSE ("true")] -> w396
                    tunnel: w398 -> [w409 _]
                    frame True {
                      n217 = Format Into String(format string="Calibration file %s is used more than once.", w409) -> (resulting string=w412:string)  [unwired: 2 in, 1 out]
                      n218 = One Button Dialog(message=w412, button name ("OK")="Ok") -> (true=w410:bool)
                    }
                    frame False {
                    }
                  }
                  n219 = Build Array (concatenate)(w402, w398) -> (w403:path[])
                  n220 = Or(x=w397, y=w396) -> (x .or. y?=w395:bool)
                }
                n221 = Or Array Elements(Boolean array=w390) -> (logical OR=w387:bool)
                n222 = Not(x=w387) -> (.not. x?=w388:bool)
              }
            }
          }
          frame #12 {
            n223 = call "Current_Calib_Filenames.vi"("Mode"=App_Global."Read Global") -> ("Calib Filename Out"=w422:path[], "Channel Numbers Out"=w423:i16[])  [unwired: 2 in, 1 out]
            n224 = for {
              tunnel: w421 -> [w436] mode=indexing
              tunnel: w423 -> [w438]
              tunnel: w422 -> [w437]
              tunnel: [w435] -> w425 mode=indexing
              w433 = Inst_type."Cross wire 2"  # Inst type
              n225 = Unbundle By Name(w436) -> ("Inst type"=w428:T2, "Ch No"=w430:i16, "Use Latest"=w431:bool, "Inst type"=w434:T2)
              n226 = Not Equal?(x=w434, y=w433) -> (x != y?=w432:bool)
              n227 = Compound Arithmetic op=AND(w431, w432) -> (w429:bool)
              n228 = Not Equal?(x=Inst_type."Raw voltage" ("Inst type"), y=w428) -> (x != y?=w426:bool)
              n229 = case shown="True" w429 {
                tunnel: w438 -> [_ w449]
                tunnel: w430 -> [_ w448]
                tunnel: w437 -> [_ w446]
                tunnel: w436 -> [w439 w445]
                tunnel: [w439 w444] -> w435
                tunnel: w426 -> [_ w441]
                frame False {
                }
                frame True {
                  n230 = Search 1D Array(1D array=w449, element=w448) -> (index of element=w447:i32)  [unwired: 1 out]
                  n231 = Index Array(array=w446, index=w447) -> (element=w442:path)
                  n232 = Select(t=w442, s=w441, f=path "") -> (s? t:f=w443:path)
                  n233 = Bundle By Name(cluster=w445, "Calib filename"=w443) -> (w444:T14)
                }
              }
            }
          }
          frame #13 {
            n234 = case shown="True" w451 {
              tunnel: w450 -> [w455 w458]
              tunnel: [w455 w457] -> w454
              tunnel: w453 -> [_ _]
              tunnel: w452 -> [_ w456]
              frame False {
              }
              frame True {
                n235 = case shown="\"Run Program\", Default" w456 {
                  tunnel: w458 -> [w460 w468]
                  tunnel: [w459 w468] -> w457
                  frame "Run Program", Default {
                    n236 = for {
                      tunnel: w460 -> [w461] mode=indexing
                      tunnel: [w462] -> w459 mode=indexing
                      n237 = Unbundle By Name(w461) -> ("Calib filename"=w467:path, "Use Latest"=w466:bool, "Ch No"=w465:i16, "Inst type"=w464:T2)
                      n238 = call "Find_calibration_file.vi"("Inst type"=w464, "Ch No"=w465, "Use Latest Calib"=w466, "filename"=w467) -> ("filename out"=w463:path)
                      n239 = Bundle By Name(cluster=w461, "Calib filename"=w463) -> (w462:T14)
                    }
                  }
                  frame "Setup Front Panel" {
                  }
                }
              }
            }
          }
          frame #14 {
            w471 = 0 ("Index")
            n240 = Index Array(array=w473, index=w471) -> (element=w472:T14)
            n241 = Initialize Array(w472, w471) -> (w470:T22)
            n242 = for {
              shift-right: [w481] -> w475
              shift-left: w470 -> [w480]
              shift-right: [w482] -> w476
              shift-left: w470 -> [w484]
              tunnel: w473 -> [w483] mode=indexing
              n243 = Unbundle By Name(w483) -> ("Move channel"=w485:bool)
              n244 = case shown="True" w485 {
                tunnel: w484 -> [w487 w493]
                tunnel: w483 -> [w489 w492]
                tunnel: [w488 w493] -> w482
                tunnel: [w486 w491] -> w481
                tunnel: w480 -> [w486 w490]
                frame False {
                  n245 = Build Array (concatenate)(w487, w489) -> (w488:T22)
                }
                frame True {
                  n246 = Build Array (concatenate)(w490, w492) -> (w491:T22)
                }
              }
            }
            n247 = Build Array (concatenate)(w476, w475) -> (w474:T22)
            n248 = for {
              tunnel: w474 -> [w479] mode=indexing
              tunnel: [w477] -> w469 mode=indexing
              n249 = Bundle By Name(cluster=w479, "Move channel"=FALSE) -> (w477:T14)
            }
          }
          frame #15 {
            n250 = Not Equal?(x=w494, y=w495) -> (x != y?=w496:bool)
            n251 = case shown="True" w496 {
              tunnel: w495 -> [_ w497]
              frame False {
              }
              frame True {
                n252 = local write "Ch & spans choices"(w497) -> ()
              }
            }
          }
          frame #16 {
            n253 = for {
              shift-right: [w507] -> _
              shift-left: string[] [] -> [w508]
              tunnel: [w510] -> w499 mode=indexing
              tunnel: [w504] -> w500 mode=indexing
              tunnel: w501 -> [w506] mode=indexing
              tunnel: [w503] -> w498 mode=indexing
              n254 = Unbundle By Name(w506) -> ("Inst type"=w509:T2)
              n255 = case shown="\"Propeller anemometer\"" w509 {
                tunnel: [w517 w521 w524 w528 w532 w536 w540 "XW" w547 w552 w555 w559] -> w504
                tunnel: ["U" "P" "U" "U" "tau" "U" "U" "W" "U" "C" "T" "T"] -> w511
                tunnel: w508 -> [w518 w522 w526 w530 w534 w538 w542 w544 w549 w553 w557 w561]
                tunnel: [w516 w520 w525 w529 w533 w537 w541 w544 w548 w551 w556 w560] -> w507
                frame "Propeller anemometer" {
                  w517 = "Prop"
                  n256 = Build Array (concatenate)(w518, w517) -> (w516:string[])
                }
                frame "Pressure Transducer" {
                  w521 = "Mano"
                  n257 = Build Array (concatenate)(w522, w521) -> (w520:string[])
                }
                frame "Raw voltage" {
                  w524 = "RV"
                  n258 = Build Array (concatenate)(w526, w524) -> (w525:string[])
                }
                frame "Pitot-static tube" {
                  w528 = "Pitot"
                  n259 = Build Array (concatenate)(w530, w528) -> (w529:string[])
                }
                frame "Preston tube" {
                  w532 = "Preston"
                  n260 = Build Array (concatenate)(w534, w532) -> (w533:string[])
                }
                frame "Hot wire" {
                  w536 = "HW"
                  n261 = Build Array (concatenate)(w538, w536) -> (w537:string[])
                }
                frame "Cross wire 1" {
                  w540 = "XW"
                  n262 = Build Array (concatenate)(w542, w540) -> (w541:string[])
                }
                frame "Cross wire 2" {
                }
                frame "Generic Linear", Default {
                  w547 = "Gen"
                  n263 = Build Array (concatenate)(w549, w547) -> (w548:string[])
                }
                frame "Fast FID" {
                  w552 = "FF"
                  n264 = Build Array (concatenate)(w553, w552) -> (w551:string[])
                }
                frame "Thermocouple" {
                  w555 = "T"
                  n265 = Build Array (concatenate)(w557, w555) -> (w556:string[])
                }
                frame "Cold wire" {
                  w559 = "CW"
                  n266 = Build Array (concatenate)(w561, w559) -> (w560:string[])
                }
              }
              n267 = call "Analyse_string_array.vi"("String array"=w507) -> ("Unique strings"=w515:string[], "Frequency"=w513:i32[])  [unwired: 1 out]
              n268 = Search 1D Array(1D array=w515, element=w504) -> (index of element=w514:i32)  [unwired: 1 out]
              n269 = Index Array(array=w513, index=w514) -> (element=w505:i32)
              n270 = Number To Decimal String(number=w505) -> (decimal integer string=w503:string)  [unwired: 1 out]
              n271 = Concatenate Strings(w503, w504, ":", w511) -> (w510:string)
            }
          }
          frame #17 {
            w570 = T8 {"Colour"=0, "Inst type"=enum."Pitot-static tube", "Inst name"="Manometer voltage", "Symbol"="U", "Code name"="", "Extra Info"="U", "Inst Array"=enum."PWA", "Index"=0, "Voltage Index"=0, "Extra Titles"=[], "Extra Values"=[]}  # Analysis info cluster
            n272 = property on="Ch Name" class="Str"() -> ("Visible"=w571:bool)  [unwired: 2 in, 2 out]
            n273 = for {
              tunnel: [w596] -> w569 mode=indexing
              tunnel: w564 -> [w593] mode=indexing
              tunnel: w567 -> [w585] mode=indexing
              tunnel: T16 {"high limit (10V)"=10.0, "low limit (-10V)"=-10.0, "Ch No"=0, "Var name"="", "Use Latest Calib"=FALSE} ("Ch and Spans") -> [w592]
              tunnel: [w591] -> w563 mode=indexing
              tunnel: w566 -> [w589] mode=indexing
              tunnel: w570 -> [w588]
              tunnel: w565 -> [w582] mode=indexing
              tunnel: w571 -> [w576]
              i -> [w572]
              n274 = Unbundle By Name(w593) -> ("Use Latest"=w586:bool, "high limit (10V)"=w595:sgl, "low limit (-10V)"=w594:sgl, "Ch No"=w587:i16, "Inst type"=w580:T2, "Symbol"=w579:string, "D"=w578:dbl, "Ch Name"=w575:string)
              n275 = Empty String/Path?(string/path=w579) -> (empty?=w583:bool)
              n276 = Select(t=w582, s=w583, f=w579) -> (s? t:f=w581:string)
              n277 = Format Into String(format string="%s (%s)" ("Format String"), w585, w581) -> (resulting string=w574:string)  [unwired: 2 in, 1 out]
              n278 = Select(t=w575, s=w576, f=w574) -> (s? t:f=w573:string)
              n279 = Bundle By Name(cluster=w592, "Use Latest Calib"=w586, "high limit (10V)"=w595, "low limit (-10V)"=w594, "Ch No"=w587, "Var name"=w573) -> (w596:T16)
              n280 = case shown="\"Propeller anemometer\", Default" w580 {
                tunnel: [w599 w602] -> w590
                tunnel: w587 -> [w597 _]
                tunnel: w578 -> [_ w600]
                frame "Propeller anemometer", Default {
                  n281 = Format Into String(format string="Ch %d" ("Format String"), w597) -> (resulting string=w599:string)  [unwired: 2 in, 1 out]
                }
                frame "Preston tube" {
                  n282 = Format Into String(format string="D = %.2f" ("Format String"), w600) -> (resulting string=w602:string)  [unwired: 2 in, 1 out]
                }
              }
              n283 = Bundle By Name(cluster=w588, "Extra Info"=w590, "Inst type"=w580, "Inst name"=w574, "Symbol"=w581, "Code name"=w589, "Inst Array"=Instrument_Array."Analogue", "Index"=w572, "Voltage Index"=w572) -> (w591:T8)
            }
            "Analysis Info cluster" <- w563
            n284 = global write "Meas_global.vi" "Ch & spans"(w569) -> ()
          }
          frame #18 {
            n285 = global read "Meas_global.vi" "Duplicate channels"() -> (w604:i32[])
            n286 = case shown="True" "Select Duplicate Channels" {
              tunnel: w607 -> [_ _]
              tunnel: w605 -> [w615 w638]
              tunnel: w604 -> [w609 w631]
              tunnel: [w608 w630] -> w603
              frame False {
                n287 = for {
                  tunnel: w615 -> [w629] mode=indexing
                  tunnel: [w628] -> w616 mode=indexing
                  n288 = Unbundle By Name(w629) -> ("Inst type"=w628:T2)
                }
                n289 = for {
                  tunnel: w609 -> [w625] mode=indexing
                  tunnel: w616 -> [w627]
                  tunnel: [w626] -> w620 mode=indexing
                  tunnel: [w625] -> w617 mode=indexing
                  n290 = Index Array(array=w627, index=w625) -> (element=w626:T2)
                }
                n291 = Array Size(array=w615) -> (size(s)=w618:i32)
                n292 = Array Max & Min(array=w620) -> (max value=w621:T2, min value=w622:T2)  [unwired: 2 out]
                n293 = Array Max & Min(array=w617) -> (max index (indices)=w619:i32)  [unwired: 3 out]
                n294 = Array Size(array=w609) -> (size(s)=w614:i32)
                n295 = Equal?(x=w621, y=w622) -> (x = y?=w624:bool)
                n296 = Greater?(x=w614, y=1) -> (0:w611:bool)
                n297 = Greater?(x=w618, y=w619) -> (0:w623:bool)
                n298 = Compound Arithmetic op=AND(w611, w624, w623) -> (w610:bool)
                n299 = Select(t=w609, s=w610, f=i32[] [] ("32bit integer")) -> (s? t:f=w608:i32[])
              }
              frame True {
                n300 = for {
                  tunnel: w638 -> [w645] mode=indexing
                  shift-right: [w640] -> w634
                  shift-left: string[] [] -> [w641]
                  tunnel: w631 -> [w643]
                  tunnel: [w639] -> w633 mode=indexing
                  i -> [w644]
                  n301 = Unbundle By Name(w645) -> ("Inst name"=w639:string)
                  n302 = Search 1D Array(1D array=w643, element=w644) -> (index of element=w642:i32)  [unwired: 1 out]
                  n303 = case shown="0, Default" w642 {
                    tunnel: w641 -> [w648 w649]
                    tunnel: w639 -> [w647 _]
                    tunnel: [w646 w649] -> w640
                    frame 0, Default {
                      n304 = Build Array (concatenate)(w648, w647) -> (w646:string[])
                    }
                    frame -1 {
                    }
                  }
                }
                n305 = call "Select_Strings.vi"("Available Ch names"=w633, "Message"="Please select similar instruments whose results columns will be combined", "Selector mode"=T17."Zero or more", "Desired Ch names (in)"=w634) -> ("Ch Indicies Choosen"=w630:i32[])  [unwired: 4 out]
                n306 = local write "Select Duplicate Channels"(FALSE ("Select Local ADAM Channels")) -> ()
              }
            }
            n307 = global write "Meas_global.vi" "Duplicate channels"(w603) -> ()
          }
          frame #19 {
            n308 = local read "XW Present?"() -> (w654:bool)
            n309 = local read "Acquisition Method"() -> (w651:T10)
            n310 = case shown="\"Take LDA data\"" "LDA data" {
              tunnel: [w666 w669] -> w656
              tunnel: w657 -> [_ w667]
              tunnel: w658 -> [_ _]
              tunnel: [w666 w668] -> w653
              frame "No LDA data" {
                w665 = FALSE  # Synchronise Analogue channels with LDA
                w666 = u8 2  # Disabled
                n311 = local write "Synchronise Analogue channels with LDA"(w665) -> ()
              }
              frame "Take LDA data" {
                n312 = stacked-sequence {
                  tunnel: [w670 _] -> w669
                  tunnel: [_ w672] -> w668
                  tunnel: w667 -> [_ w673]
                  frame #0 {
                    w670 = u8 0  # Disabled
                  }
                  frame #1 {
                    n313 = Array Size(array=w673) -> (size(s)=w674:i32)
                    n314 = Not Equal To 0?(x=w674) -> (x != 0?=w671:bool)
                    n315 = case shown="False" w671 {
                      tunnel: w671 -> [w676 _]
                      tunnel: [w675 w677] -> w672
                      frame False {
                        w675 = u8 2  # Disabled
                        n316 = local write "Synchronise Analogue channels with LDA"(w676) -> ()
                      }
                      frame True {
                        w677 = u8 0  # Disabled
                      }
                    }
                  }
                }
              }
            }
            n317 = property on="Cross wire/LDA" class="Enum (strict)"("Visible"=w654) -> ()  [unwired: 2 in, 2 out]
            n318 = case shown="True" w654 {
              tunnel: [w663 "Cross wire"] -> w652
              frame False {
                w663 = T7."2nd component as calculated"  # Cross wire/LDA
              }
              frame True {
              }
            }
            n319 = case shown="\"DT LV-link\"" w651 {
              tunnel: [T18."Enabled" ("Disabled") T18."Enabled" ("Disabled") T18."Disabled and Grayed Out" ("Disabled")] -> w650
              frame "ADC488" {
              }
              frame "DT LV-link" {
              }
              frame "Local ADAM", Default {
              }
            }
            n320 = global write "Meas_global.vi" "Cross wire + or -ve"(w652) -> ()
            n321 = property on="Trigger mode" class="Enum (strict)"("Disabled"=w650) -> ()  [unwired: 2 in, 2 out]
            n322 = Wait (ms)(milliseconds to wait=u32 100) -> ()  [unwired: 1 out]
            n323 = property on="Synchronise Analogue channels with LDA" class="Bool (strict)"("Disabled"=w653) -> ()  [unwired: 2 in, 2 out]
            n324 = property on="LDA set up" class="Clust (strict)"("Disabled"=w656) -> ()  [unwired: 2 in, 2 out]
          }
          frame #20 {
            n325 = And(x=w683, y=w684) -> (x .and. y?=w682:bool)
            n326 = local read "Synchronise Analogue channels with LDA"() -> (w681:bool)
            n327 = while {
              shift-left: _ -> [w711]
              shift-right: [w712] -> w678
              tunnel: [w713] -> w680
              stop <- FALSE continue-if-true
              n328 = local read "Setup filename selector"() -> (w712:u16)
              n329 = Not Equal?(x=w712, y=w711) -> (x != y?=w713:bool)
            }
            n330 = case shown="True" w681 {
              tunnel: w685 -> [_ w696]
              tunnel: w682 -> [_ w695]
              frame False {
              }
              frame True {
                n331 = local write "Trigger mode"(Trigger_Mode."Trigger Every Block" ("Trigger mode")) -> ()
                n332 = case shown="True" w695 {
                  tunnel: w696 -> [_ w700]
                  frame False {
                  }
                  frame True {
                    n333 = for {
                      tunnel: w700 -> [w709] mode=indexing
                      tunnel: [w702] -> w699 mode=indexing
                      n334 = Unbundle By Name(w709) -> ("Inst type"=w708:T2, "Symbol"=w706:string)
                      n335 = Equal?(x=w706, y="Sync") -> (x = y?=w704:bool)
                      n336 = Equal?(x=Inst_type."Raw voltage" ("Inst type"), y=w708) -> (x = y?=w703:bool)
                      n337 = And(x=w703, y=w704) -> (x .and. y?=w702:bool)
                    }
                    n338 = Or Array Elements(Boolean array=w699) -> (logical OR=w698:bool)
                    n339 = case shown="False" w698 {
                      frame False {
                        n340 = One Button Dialog(message="To Perform LDA Sync you must provide a Raw voltage channel having the symbol \"Sync\"") -> ()  [unwired: 2 out]
                      }
                      frame True {
                      }
                    }
                  }
                }
              }
            }
            n341 = case shown="True" w680 {
              tunnel: [FALSE ("exists?") w694] -> w679
              tunnel: w678 -> [_ w692]
              frame False {
              }
              frame True {
                n342 = local read "Setup Paths"() -> (w693:string[])
                n343 = Index Array(array=w693, index=w692) -> (element=w690:string)
                n344 = call "Setup_Filepath.vi"("Setup File Type"=Setup_Filetype."Measurement Setups", "Filename in"=w690) -> ("Filename Out"=w689:path)  [unwired: 1 out]
                n345 = call "Does_file_exist_(simple).vi"("Pathname"=w689) -> ("exists?"=w694:bool)
              }
            }
            n346 = local write "Read Setup File?"(w679) -> ()
            n347 = Current VI's Path() -> (path=w686:path)
            n348 = call "Close_Panel_and_Abort.vi"("Vi path"=w686, "stop"="stop") -> ()  [unwired: 1 out]
          }
        }
      }
    }
    frame #5 {
      n349 = local read "LDA data"() -> (w719:enum16{"No LDA data", "Take LDA data"})
      n350 = case shown="\"Take LDA data\"" w719 {
        tunnel: [FALSE ("Synchronise Analogue channels with LDA") "Synchronise Analogue channels with LDA"] -> w714
        frame "No LDA data" {
        }
        frame "Take LDA data" {
        }
      }
      n351 = global write "Meas_global.vi" "Synchronise with LDA"(w714) -> ()
      n352 = global write "Meas_global.vi" "LDA data"(w719) -> ()
      n353 = Unbundle By Name("LDA set up") -> ("dimensions"=w717:enum16{"1D", "2D"}, "Arrival spacing"=w716:bool, "Transit time"=w715:bool)
      n354 = global write "Meas_global.vi" "dimensions"(w717) -> ()
      n355 = global write "Meas_global.vi" "Arrival spacing"(w716) -> ()
      n356 = global write "Meas_global.vi" "Transit time"(w715) -> ()
    }
    frame #6 {
      n357 = stacked-sequence {
        seq-local: [_ w751 _ _] -> [_ _ _ w839]
        seq-local: [_ _ w807 _] -> [_ _ _ w838]
        seq-local: [w727 _ _ _] -> [_ _ _ w826]
        tunnel: w724 -> [w726 _ _ w830]
        tunnel: w723 -> [_ _ _ w829]
        tunnel: w722 -> [w725 _ _ _]
        frame #0 {
          n358 = local read "PWA Data"() -> (w728:T1)
          n359 = case shown="\"One Ch PWA\"" w728 {
            tunnel: ["" w737] -> w727
            tunnel: w726 -> [_ w736]
            tunnel: w725 -> [_ w732]
            frame "No PWA Data" {
            }
            frame "One Ch PWA" {
              n360 = Not Equal?(x="Calib_Setup.xls", y=w732) -> (x != y?=w731:bool)
              n361 = case shown="\"Setup Front Panel\"" w736 {
                tunnel: [w741 w744 w747 w750] -> w735
                tunnel: [w740 w743 w746 w749] -> w734
                tunnel: [w739 w742 w745 w748] -> w730
                tunnel: w731 -> [w739 w742 w745 _]
                frame "Show Setup" {
                  w741 = TRUE  # Show Panel?
                  w740 = T4 FALSE  # OK
                }
                frame "Run Program" {
                  w744 = FALSE  # Show Panel?
                  w743 = T4 TRUE  # OK
                }
                frame "Save Current Setup" {
                  w747 = FALSE  # Show Panel?
                  w746 = T4 TRUE  # OK
                }
                frame "Setup Front Panel" {
                  w748 = FALSE  # Check Calib file?
                  w750 = FALSE  # Show Panel?
                  w749 = T4 TRUE  # OK
                }
              }
              n362 = global read "Meas_global.vi" "Pre Setup String"() -> (w738:string)
              n363 = call "PWA_Setup_Panel.vi"("Show Panel?"=w735, "Check Calib file?"=w730, "OK"=w734, "Incoming Setup String"=w738) -> ("Outgoing Setup String"=w737:string)  [unwired: 3 out]
            }
          }
        }
        frame #1 {
          n364 = local read "LDA set up"() -> (w758:T6)
          n365 = global read "Meas_global.vi" "Duplicate channels"() -> (w757:i32[])
          n366 = for {
            N: 3 -> [_]
            tunnel: w758 -> [w774]
            tunnel: "LDA " ("Substring") -> [w771]
            shift-right: [w767] -> w753
            shift-left: "" -> [w768]
            i -> [w775]
            n367 = case shown="2" w775 {
              tunnel: w774 -> [w779 w785 w791]
              tunnel: [w777 w783 w789] -> w773
              tunnel: ["Dimensions" "Arrival spacing" "Transit Time"] -> w772
              frame 0, Default {
                n368 = Unbundle By Name(w779) -> ("dimensions"=w778:enum16{"1D", "2D"})
                n369 = case shown="\"2D\"" w778 {
                  tunnel: ["1D" "2D"] -> w777
                  frame "1D" {
                  }
                  frame "2D" {
                  }
                }
              }
              frame 1 {
                n370 = Unbundle By Name(w785) -> ("Arrival spacing"=w784:bool)
                n371 = case shown="False" w784 {
                  tunnel: ["FALSE" "TRUE"] -> w783
                  frame False {
                  }
                  frame True {
                  }
                }
              }
              frame 2 {
                n372 = Unbundle By Name(w791) -> ("Transit time"=w790:bool)
                n373 = case shown="False" w790 {
                  tunnel: ["FALSE" "TRUE"] -> w789
                  frame False {
                  }
                  frame True {
                  }
                }
              }
            }
            n374 = Concatenate Strings(w771, w772) -> (w770:string)
            n375 = call "Characters_to_string.vi"("Characters to write"=w773, "Label for characters"=w770) -> ("Output string"=w769:string)
            n376 = Concatenate Strings(w768, w769) -> (w767:string)
          }
          n377 = for {
            shift-right: [w762] -> w755
            shift-left: "" -> [w765]
            tunnel: w757 -> [w766] mode=indexing
            n378 = Number To Decimal String(number=w766) -> (decimal integer string=w764:string)  [unwired: 1 out]
            n379 = Concatenate Strings(w765, w764, "; ") -> (w762:string)
          }
          n380 = call "Characters_to_string.vi"("Characters to write"=w755, "Label for characters"="Log_Similar_Measurements_in_the _same_column") -> ("Output string"=w752:string)
          n381 = Concatenate Strings(w753, w752) -> (w751:string)
        }
        frame #2 {
          n382 = global write "Meas_global.vi" "Trigger mode"("Trigger mode") -> ()
          n383 = local read "Cross wire"() -> (w810:T7)
          n384 = global read "Preference_global.vi" "Rig Setup"() -> (w796:string)
          n385 = Match Pattern(string=w796, regular expression="-") -> (before substring=w795:string)  [unwired: 4 out]
          n386 = case shown="\"Free Running\"" "Trigger mode" {
            tunnel: ["Free Running" "Trigger Every Block" "Trigger Every Sample" "Start on Trigger"] -> w805
            frame "Free Running" {
            }
            frame "Trigger Every Block" {
            }
            frame "Trigger Every Sample" {
            }
            frame "Start on Trigger" {
            }
          }
          n387 = property on="PWA Data" class="Enum (strict)"() -> ("Strings []"=w801:string[])  [unwired: 2 in, 2 out]
          n388 = global write "Meas_global.vi" "PWA Data"("PWA Data") -> ()
          n389 = Equal?(x=T7."2nd component multipled by -1" ("Cross wire/LDA"), y=w810) -> (x = y?=w809:bool)
          n390 = case shown="\"EnFlo_Tunnel\"" w795 {
            tunnel: ["" w817] -> w794
            frame "False", Default {
            }
            frame "EnFlo_Tunnel" {
              n391 = call "Characters_to_string.vi"("Characters to write"="FALSE", "Label for characters"="Show_all_EnFlo_Tunnel_Columns") -> ("Output string"=w817:string)
            }
          }
          n392 = Index Array(array=w801, index="PWA Data") -> (element=w800:string)
          n393 = Select(t="TRUE", s=w809, f="FALSE") -> (s? t:f=w812:string)
          n394 = call "Characters_to_string.vi"("Characters to write"=w800, "Label for characters"="Pulsed_Wire_Data" ("Variable name")) -> ("Output string"=w799:string)
          n395 = call "Characters_to_string.vi"("Characters to write"=w812, "Label for characters"="Invert Second Component") -> ("Output string"=w808:string)
          n396 = call "Characters_to_string.vi"("Characters to write"=w805, "Label for characters"="Trigger mode") -> ("Output string"=w803:string)
          n397 = Concatenate Strings(w803, w799, w808, w794) -> (w807:string)
        }
        frame #3 {
          w831 = FALSE  # Show Panel?
          n398 = for {
            tunnel: w829 -> [w844] mode=indexing
            tunnel: [w843] -> w825 mode=indexing
            n399 = Unbundle By Name(w844) -> ("Ch Name"=w843:string)
          }
          n400 = global read "Meas_global.vi" "Pre Setup String"() -> (w832:string)
          n401 = call "Choose_Plug_In_to_Run.vi"("setup"=w830, "Show Panel?"=w831, "Setup String In"=w832) -> ("Setup String Out"=w833:string)  [unwired: 1 out]
          n402 = Array To Spreadsheet String(array=w825, 3:"%s" ("format string")) -> (spreadsheet string=w827:string)  [unwired: 1 out]
          n403 = call "Add_label_to_string.vi"("String to write"=w827, "File Label"="Local ADAM Channels") -> ("Output string"=w840:string)
          n404 = call "Date_and_Time_to_string.vi"() -> ("Date and time (spreadsheet)"=w835:string)
          n405 = global read "Meas_global.vi" "New Setup String"() -> (w834:string)
          n406 = call "Value_to_string.vi"("Value"="Sync Delay Time (ms)", "Label for value"="Sync Delay Time (ms)" ("Label for characters")) -> ("Output string"=w828:string)  [unwired: 1 in]
          n407 = Concatenate Strings(w834, w826, w833, w835, w839, w838, w840, w828) -> (w842:string)
          n408 = global write "Meas_global.vi" "New Setup String"(w842) -> ()
          n409 = global write "LDA_meas_global_1.vi" "Sync Delay Time (ms)"("Sync Delay Time (ms)") -> ()
        }
      }
    }
    frame #7 {
    }
    frame #8 {
      n410 = case shown="\"Take New Data\"" w846 {
        tunnel: w847 -> [w854 w889]
        tunnel: [w848 w883] -> w845
        frame "Take New Data" {
          n411 = for {
            tunnel: w854 -> [w865] mode=indexing
            shift-right: [w861] -> w851
            shift-left: i16[] [] -> [w863]
            shift-right: [w859] -> w850
            shift-left: path[] [] -> [w860]
            tunnel: [w856] -> w848 mode=indexing
            n412 = Unbundle By Name(w865) -> ("Use Latest"=w858:bool, "Inst type"=w864:T2, "Ch No"=w862:i16, "Calib filename"=w857:path)
            n413 = call "Current_Filepath.vi"("Filename in"=w857, "Data Type"="Calibrations") -> ("Filename Out"=w856:path)  [unwired: 1 out]
            n414 = case shown="\"Propeller anemometer\", Default" w864 {
              tunnel: w863 -> [w872 w882]
              tunnel: w862 -> [w871 _]
              tunnel: [w870 w882] -> w861
              tunnel: w860 -> [w869 w881]
              tunnel: w857 -> [w868 _]
              tunnel: [w867 w881] -> w859
              tunnel: w858 -> [w866 _]
              frame "Propeller anemometer", Default {
                n415 = case shown="False" w866 {
                  tunnel: w872 -> [w878 w880]
                  tunnel: w871 -> [w877 _]
                  tunnel: [w876 w880] -> w870
                  tunnel: w869 -> [w875 w879]
                  tunnel: w868 -> [w874 _]
                  tunnel: [w873 w879] -> w867
                  frame False {
                    n416 = Build Array (concatenate)(w878, w877) -> (w876:i16[])
                    n417 = Build Array (concatenate)(w875, w874) -> (w873:path[])
                  }
                  frame True {
                  }
                }
              }
              frame "Raw voltage" {
              }
            }
          }
          n418 = call "Current_Calib_Filenames.vi"("Calib Filename"=w850, "Channel Numbers"=w851, "Mode"=App_Global."Write to Global") -> ()  [unwired: 3 out]
        }
        frame "Post Process Raw Data File" {
          n419 = for {
            tunnel: w889 -> [w895] mode=indexing
            tunnel: [w894] -> w883 mode=indexing
            n420 = Unbundle By Name(w895) -> ("Calib filename"=w894:path)
          }
          n421 = global read "Meas_global.vi" "Pre Setup String"() -> (w888:string)
          n422 = call "Get_Characters_from_string.vi"("Input string"=w888, "Variable name"="Skip_Block_Numbers_(eg 1;2;5;12)") -> ("Status"=w886:enum16{"Char in string", "Char not in string"}, "Value"=w885:string)  [unwired: 1 in]
          n423 = case shown="\"Char in string\"" w886 {
            tunnel: w885 -> [w892 _]
            tunnel: [w890 i32[] []] -> w884
            frame "Char in string" {
              n424 = call "Get_array_values_fr_String.vi"("String Value"=w892) -> ("Numeric Array"=w891:dbl[])  [unwired: 1 out]
              n425 = To Long Integer(number=w891) -> (32bit integer=w890:i32[])
            }
            frame "Char not in string" {
            }
          }
          n426 = global write "Meas_global.vi" "Blocks to Skip"(w884) -> ()
        }
      }
      n427 = global write "Meas_global.vi" "Calib files"(w845) -> ()
    }
  }
